vi "DecodeTrame.vi"(0 "Commande":string) -> (1 "Capteur":T2=enum."Accéléromètre", 2 "Valeurs":T1)   [LabVIEW 2011]
uses:
  Capteurs.ctl
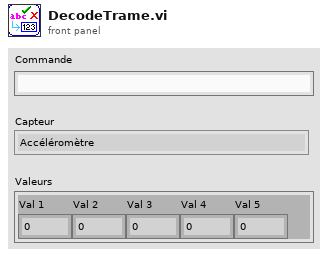
[diagram p1: front panel]
types:
  T1 = cluster{"Val 1":dbl, "Val 2":dbl, "Val 3":dbl, "Val 4":dbl, "Val 5":dbl}
  T2 = typedef "Capteurs.ctl" = enum16{"Commande invalide !", "Capteur invalide !", "Accéléromètre", "Gyroscope", "Pression", "Température", "Magnétomètre", "Altitude", "Tension accu", "Courant accu", "Angles gyroscope", "Duty cycle PWM"}
  T3 = cluster{"[0]":dbl, "[1]":dbl, "[2]":dbl, "[3]":dbl, "[4]":dbl}
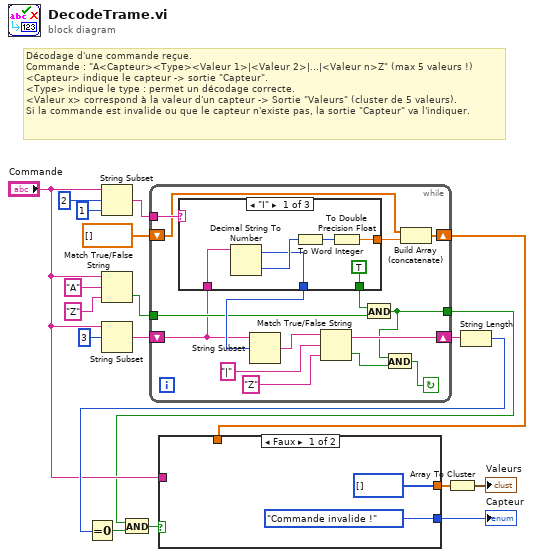
[diagram p0: block diagram]
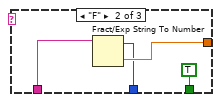
[diagram p2: hidden frame]
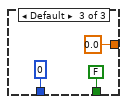
[diagram p3: hidden frame]
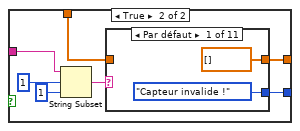
[diagram p4: hidden frame]
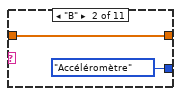
[diagram p5: hidden frame]
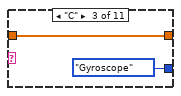
[diagram p6: hidden frame]
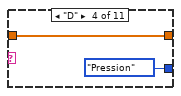
[diagram p7: hidden frame]
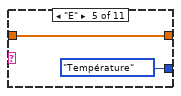
[diagram p8: hidden frame]
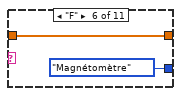
[diagram p9: hidden frame]
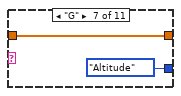
[diagram p10: hidden frame]
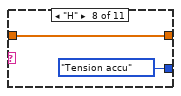
[diagram p11: hidden frame]
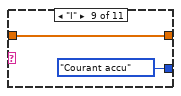
[diagram p12: hidden frame]
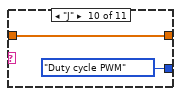
[diagram p13: hidden frame]
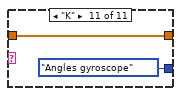
[diagram p14: hidden frame]
diagram:
  # "Décodage d'une commande reçue.\nCommande : \"A<Capteur><Type><Valeur 1>|<Valeur 2>|...|<Valeur n>Z\" (max 5 valeurs !)\n<Capteur> indique le capteur -> sortie \"Capteur\".\n<Type> indique le type : permet un décodage correcte.\n<Valeur x> correspond à la valeur d'un capteur -> Sortie \"Valeurs\" (cluster de 5 valeurs).\nSi la commande est invalide ou que le capteur n'existe pas, la sortie \"Capteur\" va l'indiquer."
  n1 = String Subset(string="Commande", offset (0)=2 ("offset"), length (rest)=1 ("valeur par défaut (0 I32)")) -> (substring=w8:string)
  n2 = Match True/False String(2:"Z" ("chaîne faux"), 3:"A" ("chaîne vrai"), 4:"Commande") -> (0:w7:bool)  [unwired: 1 out]
  n3 = String Subset(string="Commande", offset (0)=3 ("y")) -> (substring=w18:string)  [unwired: 1 in]
  n4 = while {
    shift-right: [w31] -> w17
    shift-left: w18 -> [w20]
    shift-right: [w30] -> w11
    shift-left: dbl[] [] -> [w28]
    tunnel: w8 -> [w29]
    tunnel: w7 -> [w21]
    tunnel: [w22] -> w1
    stop <- w25 continue-if-true
    n5 = case shown="\"I\"" w29 {
      tunnel: [w38 w44 0.0] -> w27
      tunnel: [w37 w43 0 ("offset past number")] -> w26
      tunnel: [TRUE TRUE FALSE] -> w23
      tunnel: w20 -> [w35 w41 _]
      frame "I" {
        n6 = Decimal String To Number(string=w35) -> (offset past number=w37:i32, number=w40:i32)  [unwired: 2 in]
        n7 = To Word Integer(number=w40) -> (16bit integer=w39:i16)
        n8 = To Double Precision Float(number=w39) -> (double precision float=w38:dbl)
      }
      frame "F" {
        n9 = Fract/Exp String To Number(string=w41) -> (offset past number=w43:i32, number=w44:dbl)  [unwired: 3 in]
      }
      frame Default {
      }
    }
    n10 = String Subset(string=w20, offset (0)=w26) -> (substring=w32:string)  [unwired: 1 in]
    n11 = Match True/False String(2:"Z" ("chaîne faux"), 3:"|" ("chaîne vrai"), 4:w32) -> (0:w24:bool, 1:w31:string)
    n12 = And(x=w23, y=w21) -> (x .and. y?=w22:bool)
    n13 = And(x=w22, y=w24) -> (x .and. y?=w25:bool)
    n14 = Build Array (concatenate)(w28, w27) -> (w30:dbl[])
  }
  n15 = String Length(string=w17) -> (length=w15:i32)
  n16 = Equal To 0?(x=w15) -> (x = 0?=w2:bool)
  n17 = And(x=w1, y=w2) -> (x .and. y?=w3:bool)
  n18 = case shown="Faux" w3 {
    tunnel: w11 -> [_ w52]
    tunnel: [Capteurs."Commande invalide !" ("CapteurEnum") w53] -> w14
    tunnel: [i16[] [] w51] -> w13
    tunnel: "Commande" -> [_ w50]
    frame False {
    }
    frame True {
      n19 = String Subset(string=w50, offset (0)=1 ("offset"), length (rest)=1 ("valeur par défaut (0 I32)")) -> (substring=w54:string)
      n20 = case shown="Par défaut" w54 {
        tunnel: [Capteurs."Capteur invalide !" ("CapteurEnum") Capteurs."Accéléromètre" ("CapteurEnum") Capteurs."Gyroscope" ("CapteurEnum") Capteurs."Pression" ("CapteurEnum") Capteurs."Température" ("CapteurEnum") Capteurs."Magnétomètre" ("CapteurEnum") Capteurs."Altitude" ("CapteurEnum") Capteurs."Tension accu" ("CapteurEnum") Capteurs."Courant accu" ("CapteurEnum") Capteurs."Duty cycle PWM" ("CapteurEnum") Capteurs."Angles gyroscope" ("CapteurEnum")] -> w53
        tunnel: w52 -> [_ w59 w61 w63 w65 w67 w69 w71 w73 w75 w77]
        tunnel: [dbl[] [] w59 w61 w63 w65 w67 w69 w71 w73 w75 w77] -> w51
        frame Default {
        }
        frame "B" {
        }
        frame "C" {
        }
        frame "D" {
        }
        frame "E" {
        }
        frame "F" {
        }
        frame "G" {
        }
        frame "H" {
        }
        frame "I" {
        }
        frame "J" {
        }
        frame "K" {
        }
      }
    }
  }
  "Capteur" <- w14
  n21 = Array To Cluster(array=w13) -> (cluster=→"Valeurs":T3)
